vi "Configure Marker Trace (Power Stat CCDF).vi"(8 "error in (no error)":errorcluster, 9 "Marker Trace (0: Measured)":i32(ring) items=["Measured", "Gaussian", "Reference"], 10 "Active Marker (1: Marker1)":i32(ring)=1 items=["Marker1"=1, "Marker2"=2, "Marker3"=3, "Marker4"=4, "Marker5"=5, "Marker6"=6, "Marker7"=7, "Marker8"=8, "Marker9"=9, "Marker10"=10, "Marker11"=11, "Marker12"=12], 11 "VISA resource name":refnum<visa-resource-name>) -> (0 "error out":errorcluster, 3 "VISA resource name out":refnum<visa-resource-name>)   [LabVIEW 2014, in "Agilent MXA Series.lvlib"]
doc: "Selects the trace that you want your marker to be placed on in Power Stat CCDF measurement type."
uses:
  Agilent MXA Series.lvlib
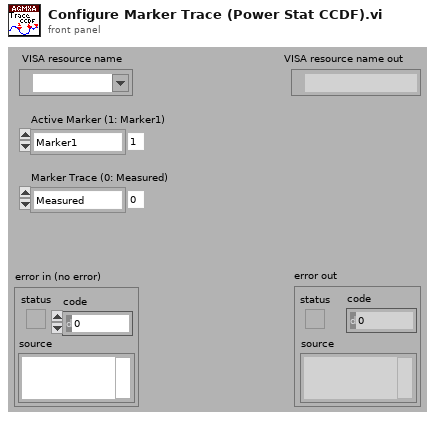
[diagram p1: front panel]
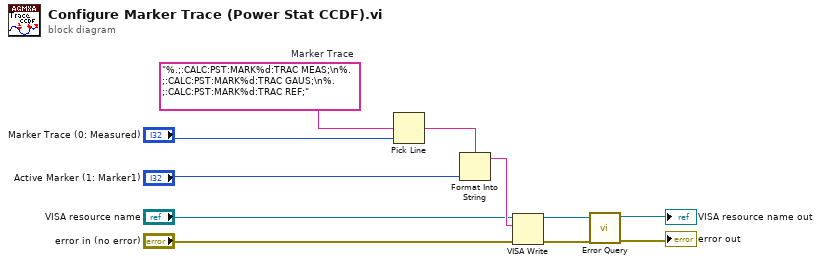
[diagram p0: block diagram]
diagram:
  w11 = "%.;:CALC:PST:MARK%d:TRAC MEAS;\n%.;:CALC:PST:MARK%d:TRAC GAUS;\n%.;:CALC:PST:MARK%d:TRAC REF;"  # Marker Trace
  n1 = Pick Line(multi-line string=w11, line index="Marker Trace (0: Measured)") -> (output string=w10:string)  [unwired: 1 in]
  n2 = Format Into String(format string=w10, "Active Marker (1: Marker1)") -> (resulting string=w7:string)  [unwired: 2 in, 1 out]
  n3 = VISA Write(VISA resource name="VISA resource name", write buffer=w7, error in (no error)="error in (no error)") -> (VISA resource name out=w4:refnum<visa-resource-name>, error out=w2:errorcluster)  [unwired: 1 out]
  n4 = call "Error Query.vi"("error in (no error)"=w2, "VISA resource name"=w4) -> ("error out"=→"error out":errorcluster, "VISA resource name out"=→"VISA resource name out":refnum<visa-resource-name>)  [unwired: 6 in, 2 out]
